vi "Keyence_写入单个寄存器数据.vi"(0 "Keyence ID In":refnum<k5>, 1 "Delay Time (s)":dbl=1.0 caption="延迟时间(s)", 5 "软元件编号":string, 9 "值":string, 11 "错误输入（无错误）":errorcluster) -> (4 "Keyence ID Out":refnum<k5>, 6 "数据输出":string, 10 "状态":bool, 15 "错误输出":errorcluster)   [LabVIEW 2017]
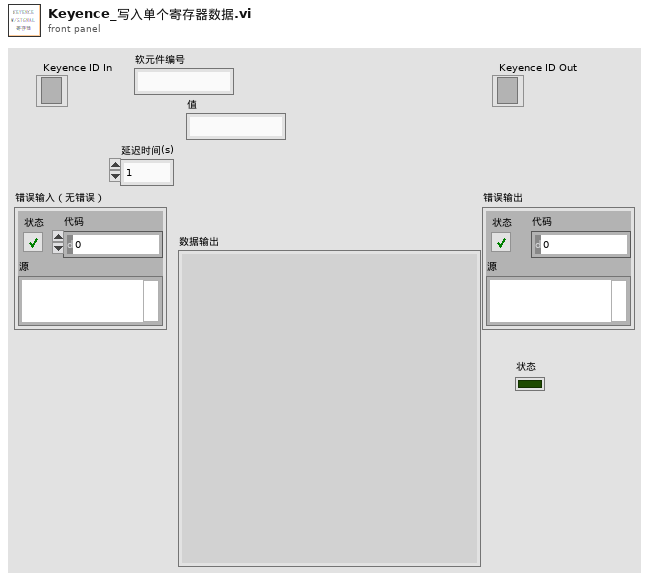
[diagram p1: front panel]
types:
  T1 = enum16{"Standard", "Buffered", "CRLF", "Immediate"}
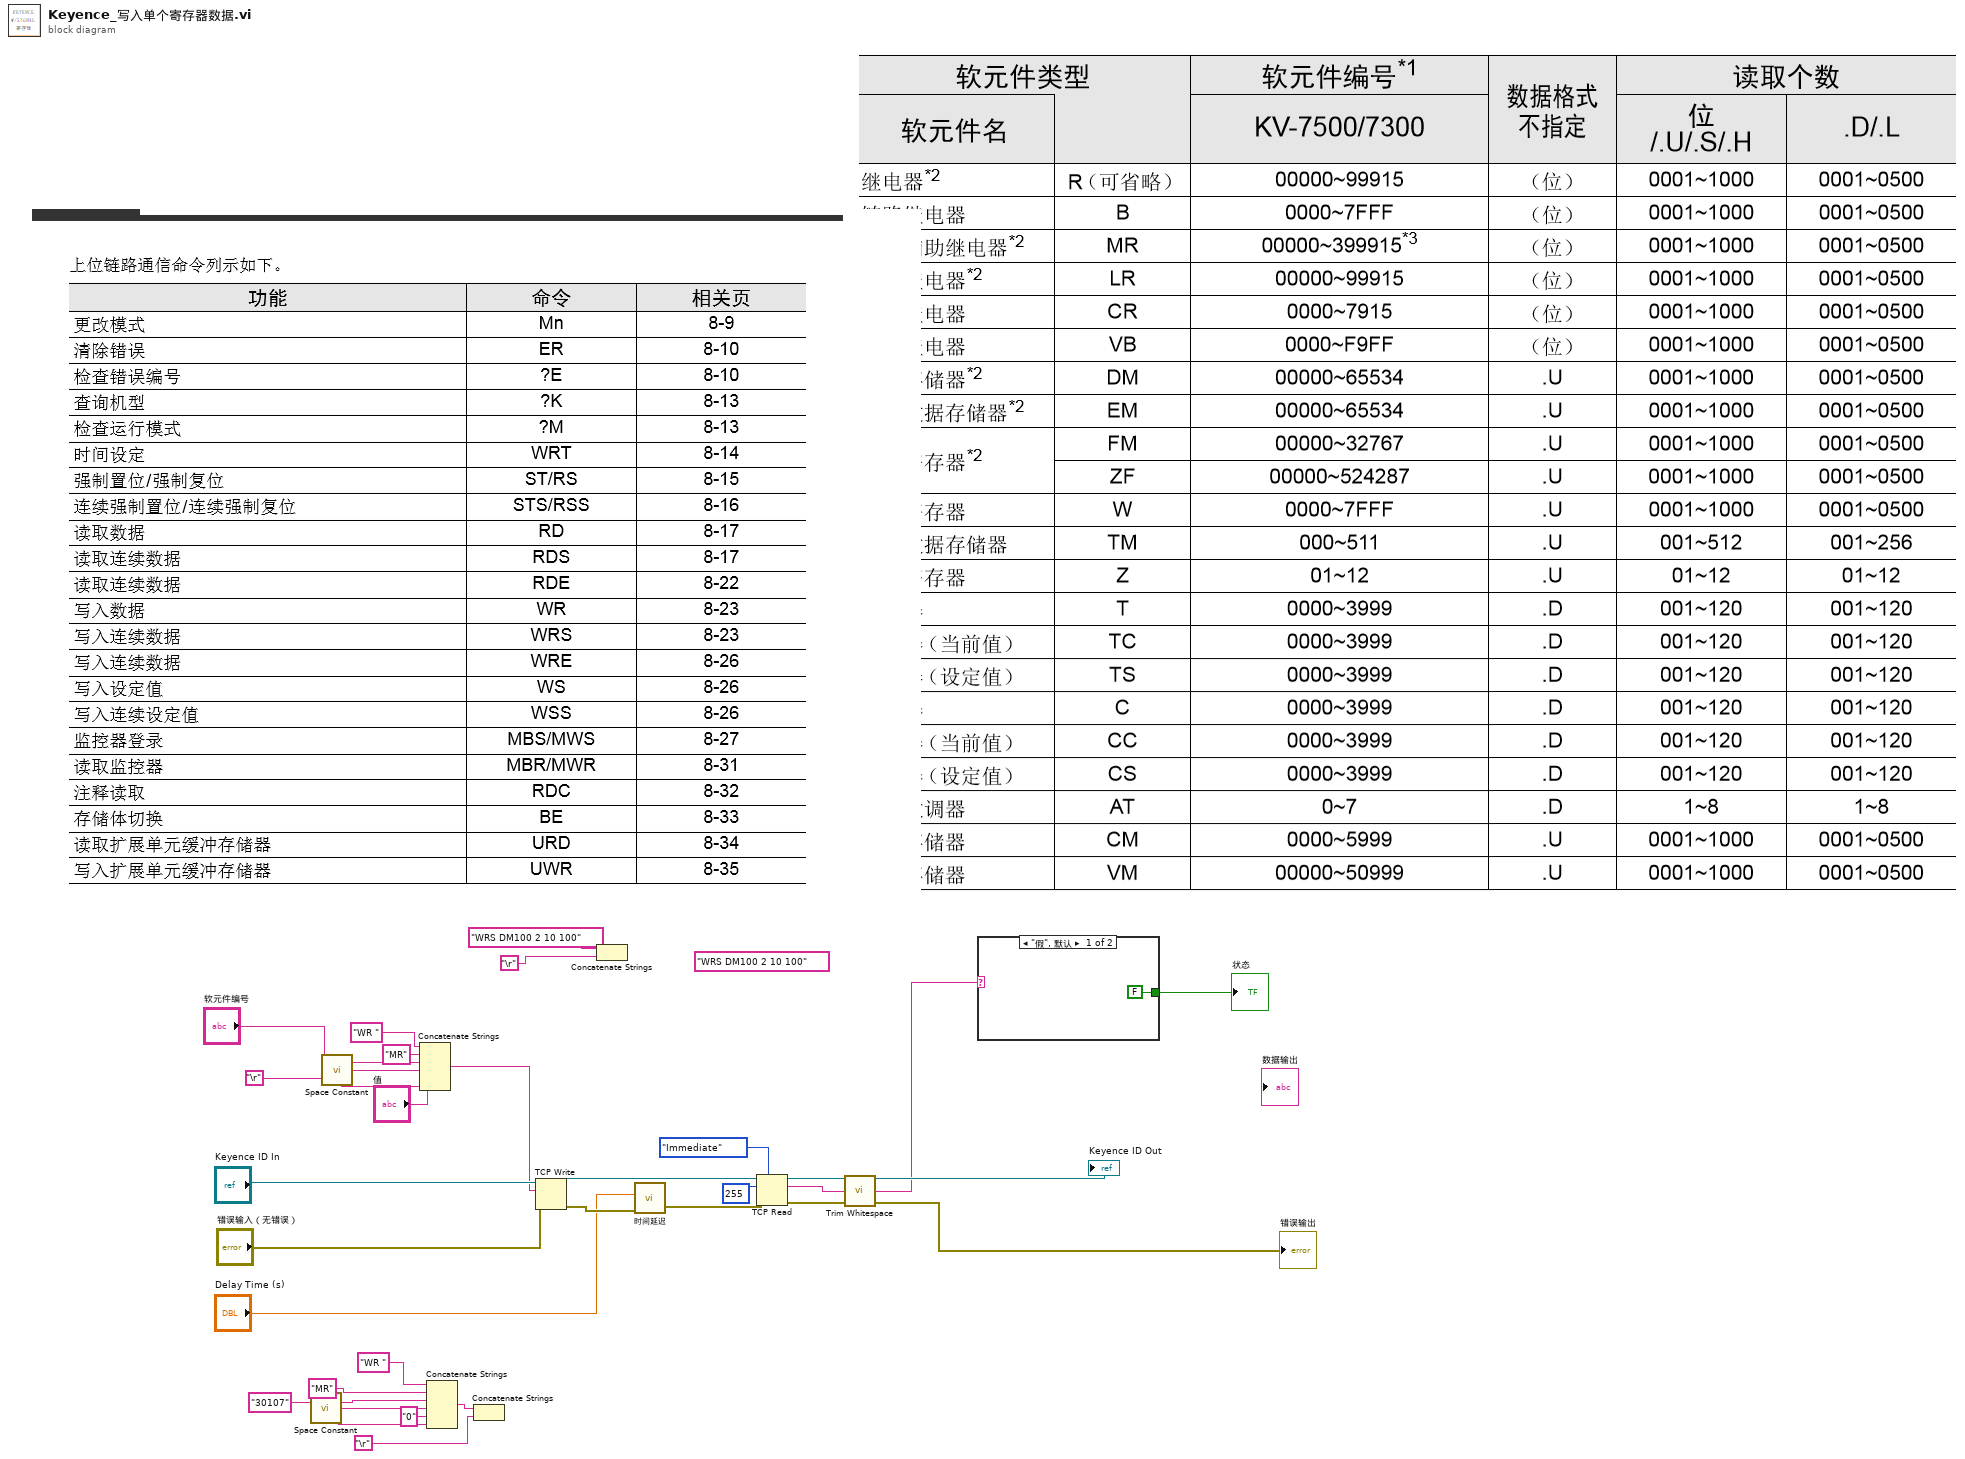
[diagram p0: block diagram]
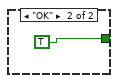
[diagram p2: hidden frame]
diagram:
  (unwired) "WRS DM100 2 10 100"
  n1 = call <vilib>:"Space Constant.vi"() -> ("String"=w4:string)
  n2 = call <vilib>:"Space Constant.vi"() -> ("String"=w16:string)
  n3 = Concatenate Strings("WR ", "MR" ("字符串"), "软元件编号", w16, "值", "\r") -> (w14:string)
  n4 = Concatenate Strings("WR ", "MR" ("字符串"), "30107" ("字符串"), w4, "0" ("字符串"), w4) -> (w3:string)
  n5 = Concatenate Strings(w3, "\r") -> ()  [unwired: 1 out]
  n6 = TCP Write(connection ID="Keyence ID In", data in=w14, error in (no error)="错误输入（无错误）") -> (connection ID out=w27:refnum<k5>, error out=w26:errorcluster)  [unwired: 1 in, 1 out]
  n7 = Concatenate Strings("WRS DM100 2 10 100", "\r") -> ()  [unwired: 1 out]
  n8 = call "时间延迟"("error in (no error)"=w26, "Delay Time (s)"="Delay Time (s)") -> ("error out"=w21:errorcluster)  [unwired: 9 in]
  n9 = TCP Read(connection ID=w27, bytes to read=255 ("读取的字节"), error in (no error)=w21, 7:T1."Immediate" ("模式（标准）")) -> (connection ID out=→"Keyence ID Out":refnum<k5>, data out=w11:string, error out=→"错误输出":errorcluster)  [unwired: 1 in]
  n10 = call <vilib>:"Trim Whitespace.vi"("string"=w11) -> ("trimmed string"=w10:string)  [unwired: 1 in]
  n11 = case shown="\"假\", 默认" w10 {
    tunnel: [FALSE TRUE] -> w9
    frame "假", Default {
    }
    frame "OK" {
    }
  }
  "状态" <- w9
